vi "Test1.vi"() -> ()   [LabVIEW 2017]
uses:
  Documents/LabVIEW Data/MathScriptVIs/MCStatic_38590875332_dd8736b7dd596d2a03d755f2a3cd6c8b.vi
  <instcachedir>/0/MCStatic_38590875332_dd8736b7dd596d2a03d755f2a3cd6c8b_DE016D958C104F27ABE4BC23A251F758.lvgen/MCStatic_38590875332_dd8736b7dd596d2a03d755f2a3cd6c8b_DE016D958C104F27ABE4BC23A251F758_000.vi
  <vilib>/imath/engines/lvmath2/RunTimeEngine/NodeEndStatement/NIMS_NodeEndStatement_Output.vi
  <instcachedir>/0/NIMS_NodeEndStatement_Output_53EC0D466D134D7ABD903AC30B43404B.lvgen/NIMS_NodeEndStatement_Output_53EC0D466D134D7ABD903AC30B43404B_001.vi
  <vilib>/imath/engines/lvmath2/RunTimeEngine/ErrorHandling/NIMS_Finalize Error.vi
  Documents/LabVIEW Data/reactor_power.m
  Documents/LabVIEW Data/control_rod_drop.m
  Documents/LabVIEW Data/long_term_power.m
  Documents/LabVIEW Data/power_function.m
  Documents/LabVIEW Data/rhoT.m
panel:
  out "Power":dbl
  out "Reactivity":dbl
  out "Reactivity rod":dbl
  out "k rod":dbl
  in  "Coolant Temp":dbl(slide) scale=0.0..200.0
  in  "Fuel Temp":dbl(slide) scale=0.0..200.0
  out "Numeric 4":dbl
  out "Numeric 3":dbl
  out "Numeric 2":dbl
  out "Waveform Chart":dbl(graph)
  out "Time":dbl
  in  "stop":bool
  in  "Soft 3":dbl(slide) scale=0.0..100.0
  in  "Soft 2":dbl(slide) scale=0.0..100.0
  in  "Soft 1":dbl(slide) scale=0.0..100.0
  in  "Med 3":dbl(slide) scale=0.0..100.0
  in  "Med 2":dbl(slide) scale=0.0..100.0
  in  "Med 1":dbl(slide) scale=0.0..100.0
  in  "Hard 3":dbl(slide) scale=0.0..100.0
  in  "Hard 2":dbl(slide) scale=0.0..100.0
  in  "Hard 1":dbl(slide) scale=0.0..100.0
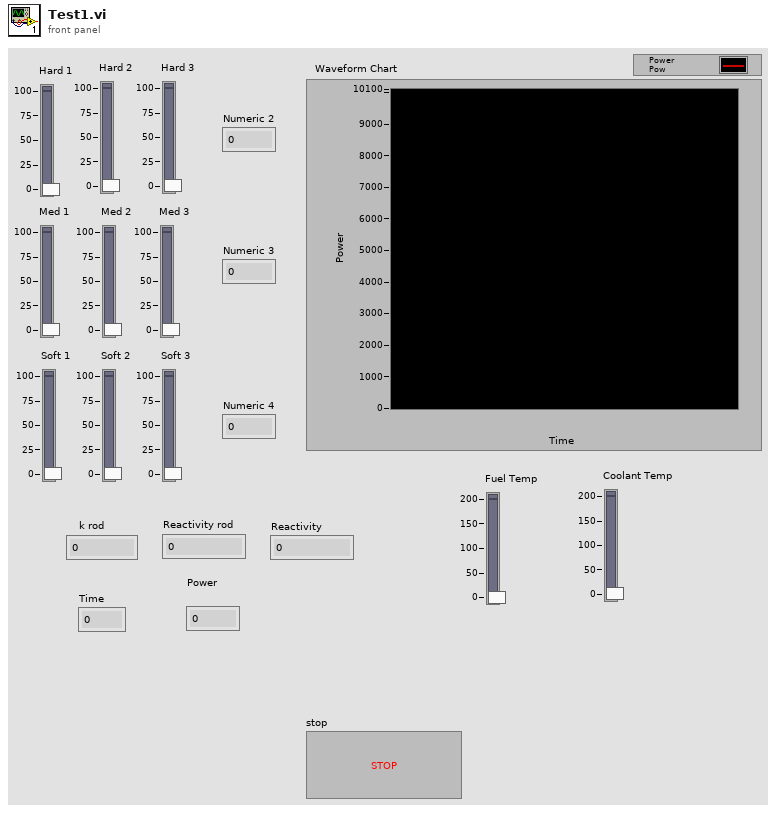
[diagram p1: front panel]
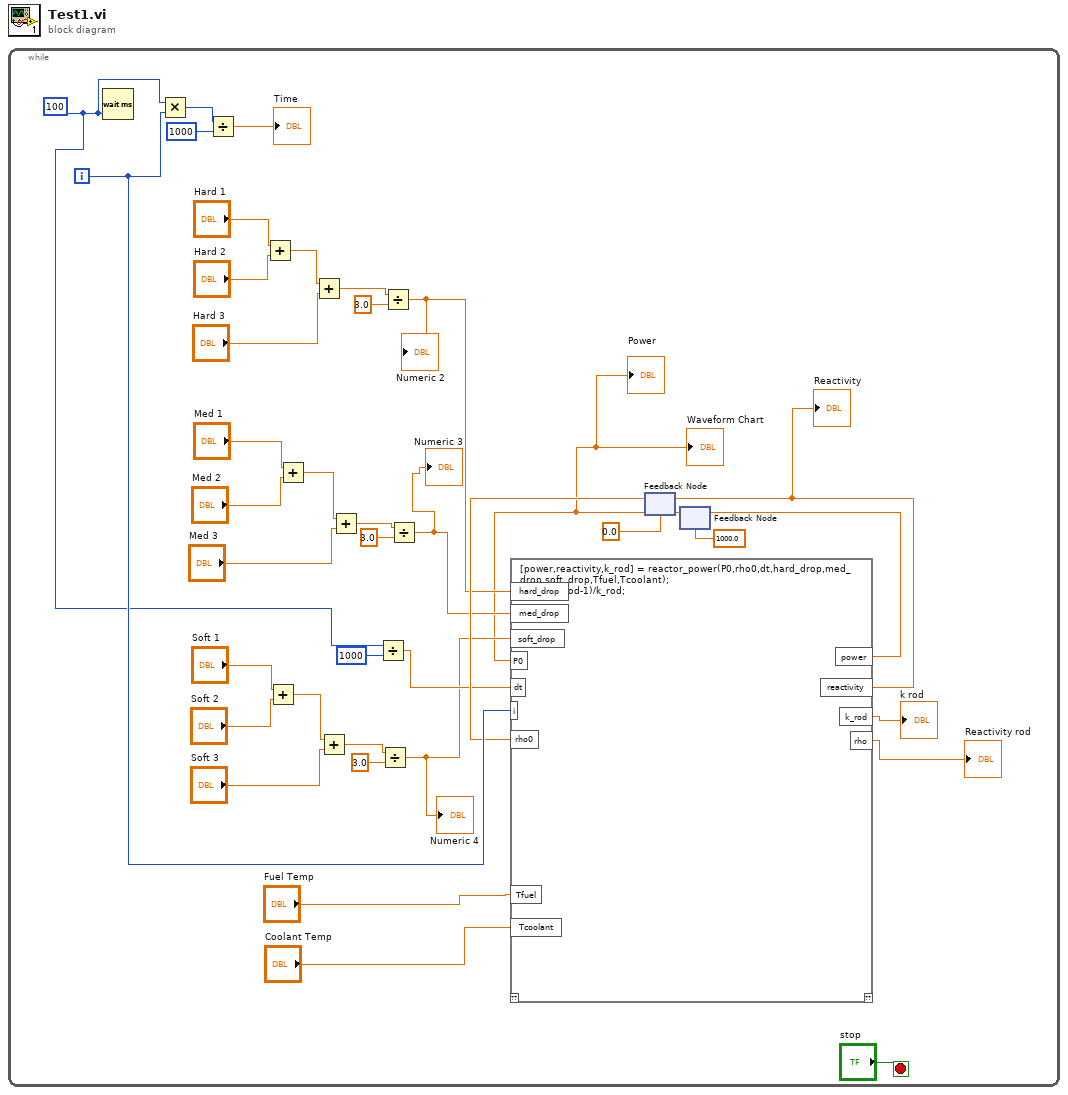
[diagram p0: block diagram]
diagram:
  n1 = while {
    i -> [w17]
    stop <- "stop" stop-if-true
    w12 = u32 100 ("milliseconds to wait")
    n2 = Wait (ms)(milliseconds to wait=w12) -> ()  [unwired: 1 out]
    n3 = Multiply(x=w12, y=w17) -> (x*y=w20:u32)
    n4 = Divide(x=w20, y=u32 1000) -> (x/y=→"Time":dbl)
    n5 = Add(x="Hard 1", y="Hard 2") -> (x+y=w35:dbl)
    n6 = Add(x="Soft 1", y="Soft 2") -> (x+y=w29:dbl)
    n7 = Add(x="Med 1", y="Med 2") -> (x+y=w23:dbl)
    n8 = Add(x=w35, y="Hard 3") -> (x+y=w34:dbl)
    n9 = Add(x=w29, y="Soft 3") -> (x+y=w28:dbl)
    n10 = Add(x=w23, y="Med 3") -> (x+y=w22:dbl)
    n11 = Divide(x=w12, y=u32 1000) -> (x/y=w10:dbl)
    n12 = Divide(x=w28, y=3.0) -> (x/y=w9:dbl)
    "Numeric 4" <- w9
    n13 = Divide(x=w34, y=3.0) -> (x/y=w7:dbl)
    "Numeric 2" <- w7
    n14 = Divide(x=w22, y=3.0) -> (x/y=w8:dbl)
    "Numeric 3" <- w8
    n15 = feedback #1(0.0 ("reactivity")) -> (w15:dbl)
    n16 = feedback #2(1000.0 ("power")) -> (w1:dbl)
    "Waveform Chart" <- w1
    "Power" <- w1
    n17 = mathscript code="[power,reactivity,k_rod] = reactor_power(P0,rho0,dt,hard_drop,med_drop,soft_drop,Tfuel,Tcoolant);\nrho = (k_rod-1)/k_rod;"("hard_drop"=w7, "med_drop"=w8, "soft_drop"=w9, "P0"=w1, "dt"=w10, "i"=w17, "rho0"=w15, "Tfuel"="Fuel Temp", "Tcoolant"="Coolant Temp") -> ("power"=w16:dbl, "reactivity"=w4:dbl, "k_rod"=→"k rod":dbl, "rho"=→"Reactivity rod":dbl)  [unwired: 1 in, 1 out]
    "Reactivity" <- w4
    n18 = feedback-in #1(w4) -> ()
    n19 = feedback-in #2(w16) -> ()
  }
